vi "piezoRun.vi"() -> ()   [LabVIEW 2017]
uses:
  <vilib>/Analysis/baseanly.llb/Mean.vi
  <vilib>/Analysis/baseanly.llb/Mean (DBL).vi
  globalUtilities.vi
  globalDevices.vi
  <userlib>/Hamamatsu Video Capture/tm_startcapture_40.vi
  <userlib>/Hamamatsu Video Capture/tm_waitnextframe_40.vi
  <userlib>/Hamamatsu Video Capture/tm_getframe16_40.vi
  <userlib>/Hamamatsu Video Capture/tm_stopcapture_40.vi
panel:
  out "Waveform Graph":dbl[](graph)
  in  "piezoWriteFunctionType":u16(ring) items=["triangle", "sine"]
  in  "stop":bool
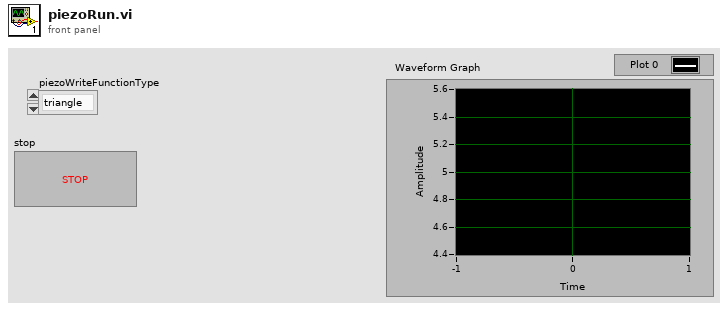
[diagram p1: front panel]
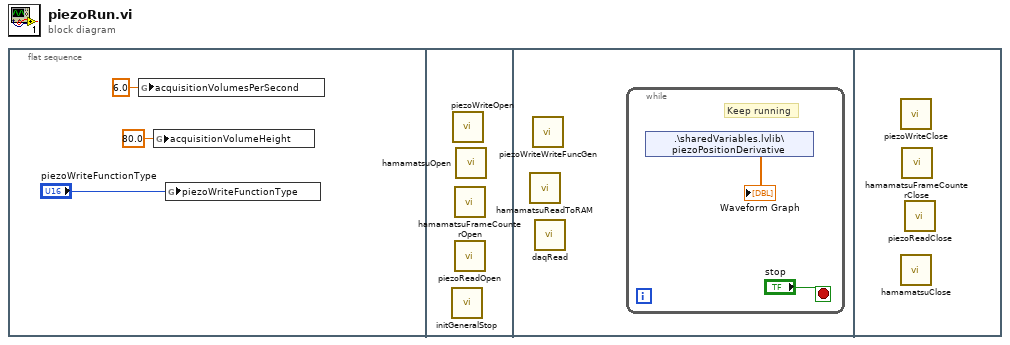
[diagram p0: block diagram]
diagram:
  n1 = flat-sequence {
    frame #0 {
      n2 = global write "globalUtilities.vi" "acquisitionVolumesPerSecond"(6.0 ("acquisitionVolumesPerSecond")) -> ()
      n3 = global write "globalUtilities.vi" "acquisitionVolumeHeight"(80.0 ("acquisitionVolumeHeight")) -> ()
      n4 = global write "globalDevices.vi" "piezoWriteFunctionType"("piezoWriteFunctionType") -> ()
    }
    frame #1 {
      n5 = call "initGeneralStop.vi"() -> ()  [unwired: 1 in]
      n6 = call "piezoWriteOpen.vi"() -> ()  [unwired: 2 in]
      n7 = call "hamamatsuFrameCounterOpen.vi"() -> ()  [unwired: 12 in]
      n8 = call "piezoReadOpen.vi"() -> ()  [unwired: 6 in]
      n9 = call "hamamatsuOpen.vi"() -> ()  [unwired: 4 out]
    }
    frame #2 {
      n10 = call "hamamatsuReadToRAM.vi"() -> ()  [unwired: 1 in, 3 out]
      n11 = call "piezoWriteWriteFuncGen.vi"() -> ()  [unwired: 12 in]
      n12 = call "daqRead.vi"() -> ()  [unwired: 3 in]
      n13 = while {
        stop <- "stop" stop-if-true
        # "Keep running"
        n14 = shared-variable ".\\sharedVariables.lvlib\\piezoPositionDerivative"() -> (→"Waveform Graph":dbl[])  [unwired: 1 in, 1 out]
      }
    }
    frame #3 {
      n15 = call "piezoWriteClose.vi"() -> ()  [unwired: 1 in]
      n16 = call "hamamatsuClose.vi"() -> ()  [unwired: 1 out]
      n17 = call "hamamatsuFrameCounterClose.vi"() -> ()  [unwired: 12 in]
      n18 = call "piezoReadClose.vi"() -> ()  [unwired: 1 in]
    }
  }
